vi "Initiate.vi"(8 "error in (no error)":errorcluster) -> (0 "error out":errorcluster, 3 "Simulation Interface out":refnum<class "Simulation Interface.lvclass">)   [LabVIEW 2013, in "Simulation Interface.lvclass"]
uses:
  Simulation Interface.lvclass
  Car Wash Controller.lvclass
  Entry Console.lvclass
  Vehicle Position Simulation.lvclass
  Wash Display Console.lvclass
  Database.lvclass
  Error Handler.lvclass
  EH Action.ctl
  Thread.lvclass
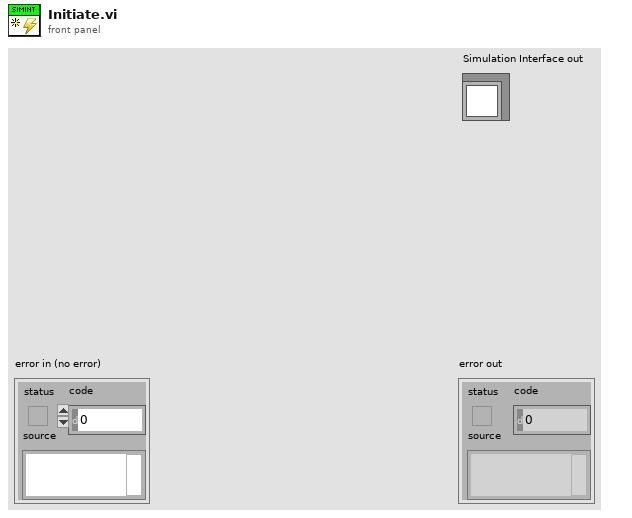
[diagram p1: front panel]
types:
  T1 = typedef "Architecture.lvlib/Error Handler.lvclass/EH Action.ctl" = enum16{"Define Threads", "Close", "System Error", "Wash Cycle Error", "Minor Error", "Initialize"}
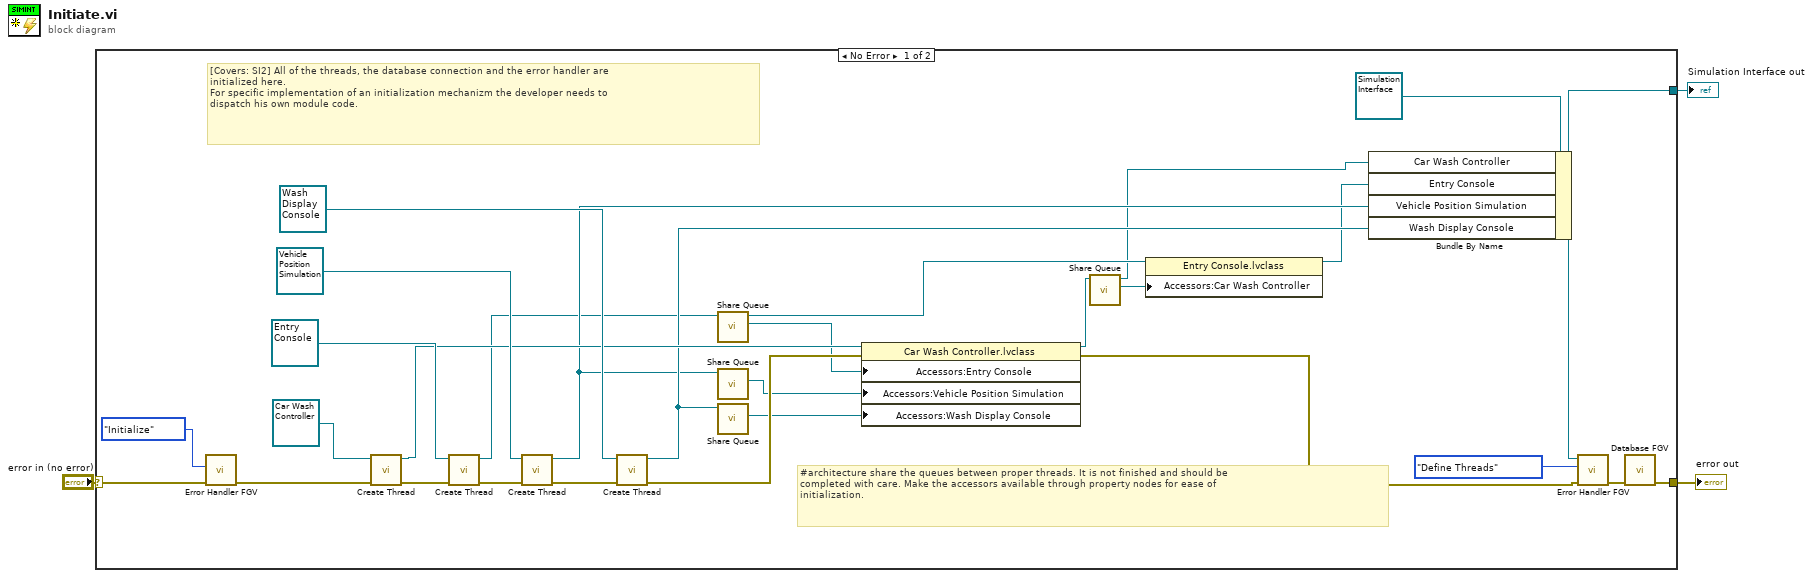
[diagram p0: block diagram]
diagram:
  n1 = case shown="No Error" "error in (no error)" {
    selector: "error in (no error)" -> [w23 w33]
    tunnel: [w24 w33] -> w2
    tunnel: [w18 _] -> w1
    frame No Error {
      # "#architecture share the queues between proper threads. It is not finished and should be \ncompleted with care. Make the accessors available through property nodes for ease of\ninitialization."
      # "[Covers: SI2] All of the threads, the database connection and the error handler are\ninitialized here.\nFor specific implementation of an initialization mechanizm the developer needs to\ndispatch his own module code."
      n2 = call "Error Handler FGV.vi"("error in (no error)"=w23, "Action"=EH_Action."Initialize") -> ("error out"=w22:errorcluster)  [unwired: 9 in]
      n3 = call-dynamic "Create Thread.vi"("error in (no error)"=w22, "Thread in"=refnum<class "Car Wash Controller.lvclass"> refnum ("Car Wash Controller.lvlib:Car Wash Controller.lvclass")) -> ("error out"=w31:errorcluster, "Thread out"=w17:refnum<class "Car Wash Controller.lvclass">)  [unwired: 8 in]
      n4 = call-dynamic "Create Thread.vi"("error in (no error)"=w31, "Thread in"=refnum<class "Entry Console.lvclass"> refnum ("Entry Console.lvlib:Entry Console.lvclass")) -> ("error out"=w30:errorcluster, "Thread out"=w9:refnum<class "Entry Console.lvclass">)  [unwired: 8 in]
      n5 = call-dynamic "Create Thread.vi"("error in (no error)"=w30, "Thread in"=refnum<class "Vehicle Position Simulation.lvclass"> refnum ("Vehicle Position Simulation.lvlib:Vehicle Position Simulation.lvclass")) -> ("error out"=w29:errorcluster, "Thread out"=w11:refnum<class "Vehicle Position Simulation.lvclass">)  [unwired: 8 in]
      n6 = call-dynamic "Create Thread.vi"("error in (no error)"=w29, "Thread in"=refnum<class "Wash Display Console.lvclass"> refnum ("Wash Display Console.lvlib:Wash Display Console.lvclass")) -> ("error out"=w16:errorcluster, "Thread out"=w14:refnum<class "Wash Display Console.lvclass">)  [unwired: 8 in]
      n7 = call "Share Queue.vi"("Thread in"=w9) -> ("Architecture.lvlib:Queue.lvclass"=w10:refnum<class "Queue.lvclass">, "Thread out"=w8:refnum<class "Entry Console.lvclass">)  [unwired: 8 in, 1 out]
      n8 = call "Share Queue.vi"("Thread in"=w11) -> ("Architecture.lvlib:Queue.lvclass"=w12:refnum<class "Queue.lvclass">)  [unwired: 8 in, 2 out]
      n9 = call "Share Queue.vi"("Thread in"=w14) -> ("Architecture.lvlib:Queue.lvclass"=w13:refnum<class "Queue.lvclass">)  [unwired: 8 in, 2 out]
      n10 = property class="Car Wash Controller.lvclass"(reference=w17, error in=w16, "Accessors:Entry Console"=w10, "Accessors:Vehicle Position Simulation"=w12, "Accessors:Wash Display Console"=w13) -> (reference out=w7:refnum<class "Car Wash Controller.lvclass">, error out=w15:errorcluster)
      n11 = call "Share Queue.vi"("Thread in"=w7) -> ("Architecture.lvlib:Queue.lvclass"=w6:refnum<class "Queue.lvclass">, "Thread out"=w5:refnum<class "Car Wash Controller.lvclass">)  [unwired: 8 in, 1 out]
      n12 = property class="Entry Console.lvclass"(reference=w8, "Accessors:Car Wash Controller"=w6) -> (reference out=w4:refnum<class "Entry Console.lvclass">)  [unwired: 1 in, 1 out]
      n13 = Bundle By Name(cluster=refnum<class "Simulation Interface.lvclass"> refnum ("Simulation Interface.lvclass"), "Car Wash Controller"=w5, "Entry Console"=w4, "Vehicle Position Simulation"=w11, "Wash Display Console"=w14) -> (w18:refnum<class "Simulation Interface.lvclass">)
      n14 = call "Error Handler FGV.vi"("error in (no error)"=w15, "Action"=EH_Action."Define Threads", "Application to EH"=w18) -> ("error out"=w19:errorcluster)  [unwired: 8 in]
      n15 = call "Database FGV.vi"("error in (no error)"=w19) -> ("error out"=w24:errorcluster)  [unwired: 8 in, 2 out]
    }
    frame Error {
    }
  }
  "error out" <- w2
  "Simulation Interface out" <- w1
